vi "Read Marker.vi"(0 "VISA resource name":refnum<visa-resource-name>, 5 "Measurement Type (6: Phase Noise)":u16(ring)=6 items=["AM Noise"=1, "Baseband Noise"=2, "Freq/Power"=3, "Spectrum"=4, "Transient"=5, "Phase Noise"=6, "User"=7], 7 "Select Trace (1: 1)":u16(ring)=1 items=["1"=1, "2"=2, "3"=3, "4"=4, "5"=5, "6"=6, "7"=7, "8"=8], 9 "Select Marker (1: 1)":u16(ring)=1 items=["1"=1, "2"=2, "3"=3, "4"=4, "5"=5, "6"=6, "7"=7, "8"=8, "9"=9, "10"=10], 11 "error in (no error)":errorcluster, 12 "Maximum Time (10000 ms)":u32=10000) -> (4 "VISA resource name out":refnum<visa-resource-name>, 6 "X Position":dbl format="%^#_9g", 10 "Y Position":dbl format="%^#_9g", 15 "error out":errorcluster)   [LabVIEW 2011, in "Agilent E5052X.lvlib"]
doc: "Reads the X and Y positions of the selected marker for the selected trace of the selected measurement. \n\n<b>Note: </b> \n\n\"Configure Marker\" and \"Configure Marker Search\" VIs should be run before calling this VI."
uses:
  Agilent E5052X.lvlib
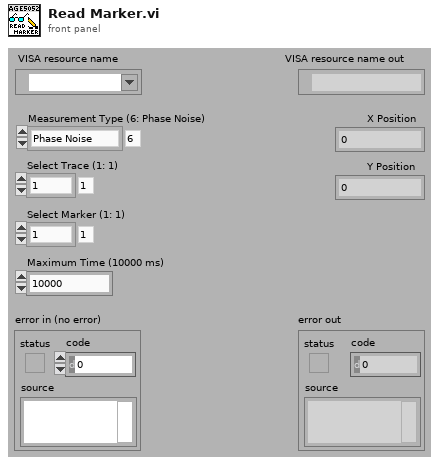
[diagram p1: front panel]
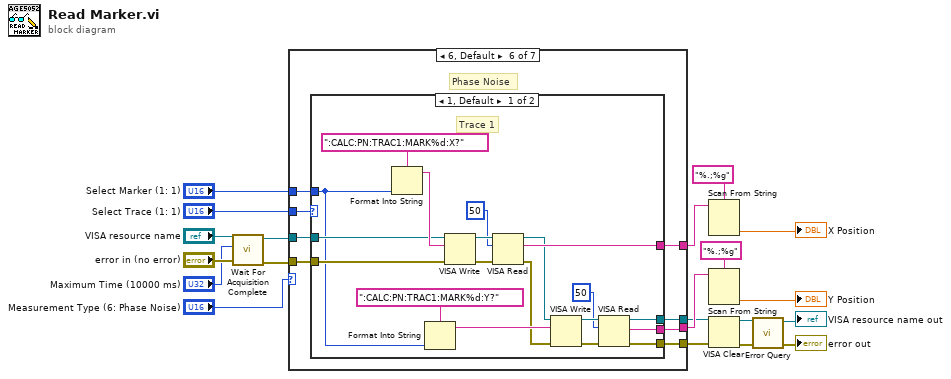
[diagram p0: block diagram]
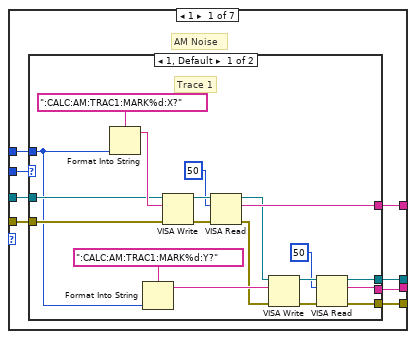
[diagram p2: hidden frame]
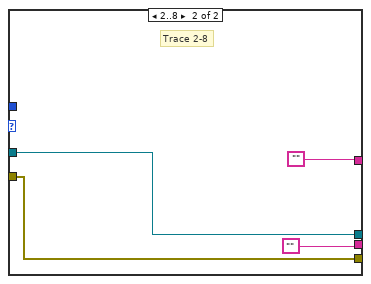
[diagram p3: hidden frame]
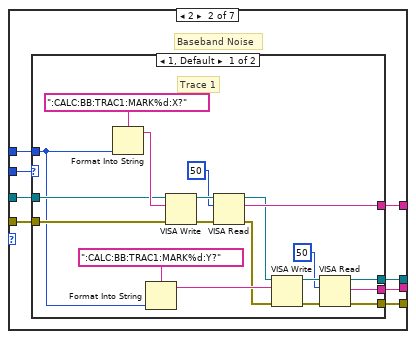
[diagram p4: hidden frame]
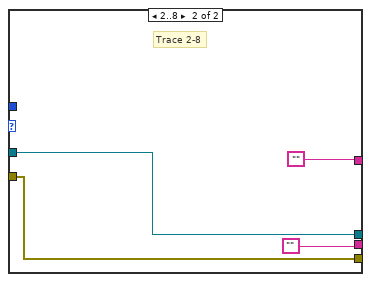
[diagram p5: hidden frame]
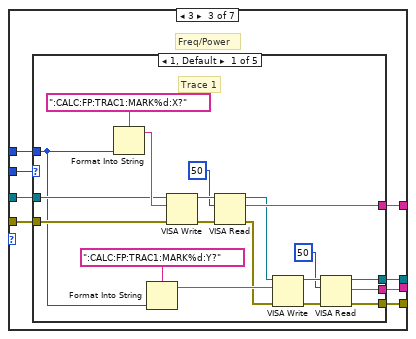
[diagram p6: hidden frame]
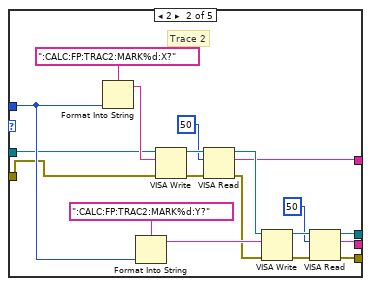
[diagram p7: hidden frame]
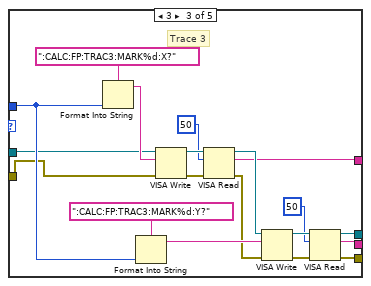
[diagram p8: hidden frame]
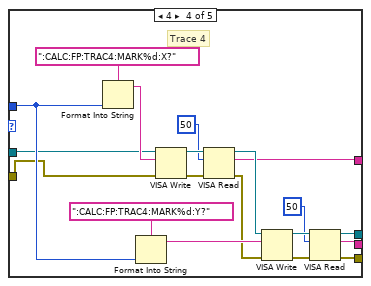
[diagram p9: hidden frame]
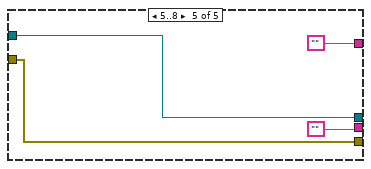
[diagram p10: hidden frame]
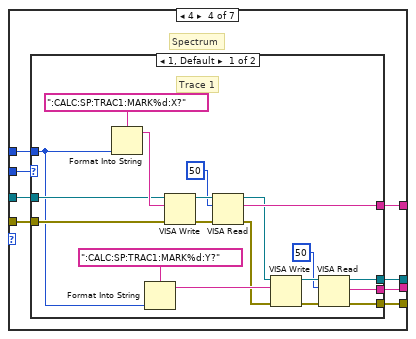
[diagram p11: hidden frame]
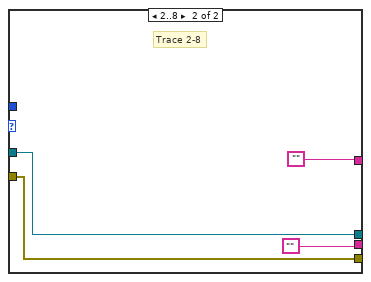
[diagram p12: hidden frame]
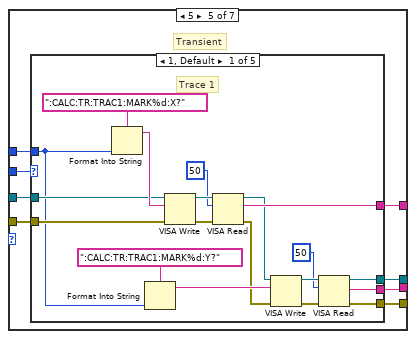
[diagram p13: hidden frame]
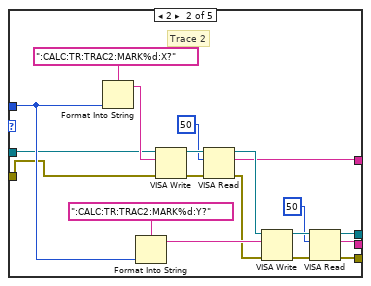
[diagram p14: hidden frame]
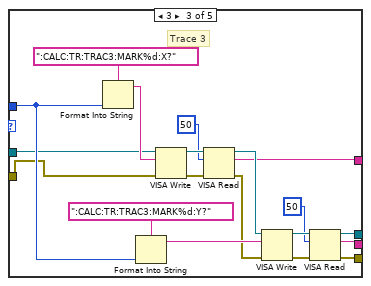
[diagram p15: hidden frame]
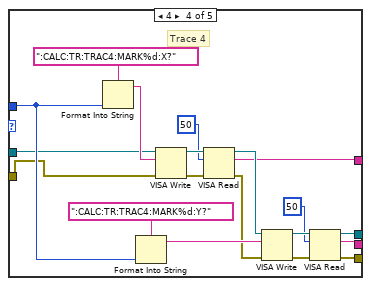
[diagram p16: hidden frame]
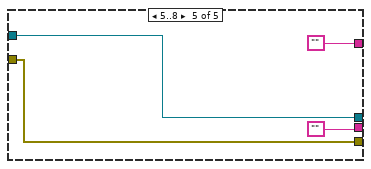
[diagram p17: hidden frame]
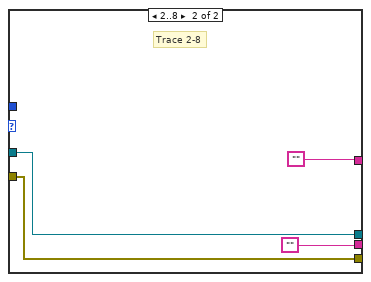
[diagram p18: hidden frame]
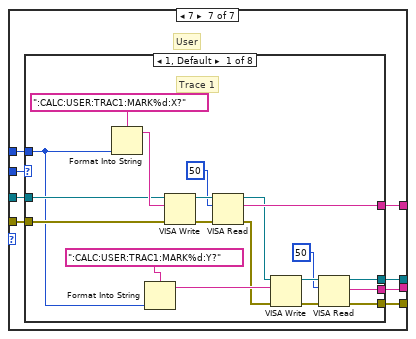
[diagram p19: hidden frame]
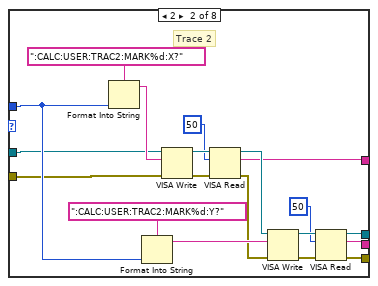
[diagram p20: hidden frame]
diagram:
  n1 = call "Wait For Acquisition Complete.vi"("error in (no error)"="error in (no error)", "Maximum Time (10000)"="Maximum Time (10000 ms)", "VISA resource name"="VISA resource name") -> ("error out"=w7:errorcluster, "VISA resource name out"=w6:refnum<visa-resource-name>)  [unwired: 7 in]
  n2 = case shown="6, Default" "Measurement Type (6: Phase Noise)" {
    tunnel: "Select Trace (1: 1)" -> [w28 w58 w89 w177 w208 w296 w327]
    tunnel: "Select Marker (1: 1)" -> [w27 w59 w90 w178 w209 w297 w328]
    tunnel: w6 -> [w26 w57 w88 w176 w207 w295 w326]
    tunnel: w7 -> [w25 w56 w87 w175 w206 w294 w325]
    tunnel: [w24 w55 w86 w174 w205 w293 w324] -> w18
    tunnel: [w23 w54 w85 w173 w204 w292 w323] -> w11
    tunnel: [w22 w53 w84 w172 w203 w291 w322] -> w15
    tunnel: [w21 w52 w83 w171 w202 w290 w321] -> w10
    frame 1 {
      # "AM Noise"
      n3 = case shown="1, Default" w28 {
        tunnel: w27 -> [w32 _]
        tunnel: w26 -> [w45 w49]
        tunnel: w25 -> [w44 w48]
        tunnel: [w40 ""] -> w24
        tunnel: [w31 w49] -> w23
        tunnel: [w30 ""] -> w22
        tunnel: [w29 w48] -> w21
        frame 1, Default {
          # "Trace 1"
          n4 = Format Into String(format string=":CALC:AM:TRAC1:MARK%d:X?", w32) -> (resulting string=w46:string)  [unwired: 2 in, 1 out]
          n5 = Format Into String(format string=":CALC:AM:TRAC1:MARK%d:Y?", w32) -> (resulting string=w38:string)  [unwired: 2 in, 1 out]
          n6 = VISA Write(VISA resource name=w45, write buffer=w46, error in (no error)=w44) -> (VISA resource name out=w42:refnum<visa-resource-name>, error out=w43:errorcluster)  [unwired: 1 out]
          n7 = VISA Read(VISA resource name=w42, byte count=u32 50, error in (no error)=w43) -> (VISA resource name out=w34:refnum<visa-resource-name>, read buffer=w40:string, error out=w33:errorcluster)  [unwired: 1 out]
          n8 = VISA Write(VISA resource name=w34, write buffer=w38, error in (no error)=w33) -> (VISA resource name out=w36:refnum<visa-resource-name>, error out=w37:errorcluster)  [unwired: 1 out]
          n9 = VISA Read(VISA resource name=w36, byte count=u32 50, error in (no error)=w37) -> (VISA resource name out=w31:refnum<visa-resource-name>, read buffer=w30:string, error out=w29:errorcluster)  [unwired: 1 out]
        }
        frame 2..8 {
          # "Trace 2-8"
        }
      }
    }
    frame 2 {
      # "Baseband Noise"
      n10 = case shown="1, Default" w58 {
        tunnel: w59 -> [w63 _]
        tunnel: w57 -> [w76 w80]
        tunnel: w56 -> [w75 w79]
        tunnel: [w71 ""] -> w55
        tunnel: [w62 w80] -> w54
        tunnel: [w61 ""] -> w53
        tunnel: [w60 w79] -> w52
        frame 1, Default {
          # "Trace 1"
          n11 = Format Into String(format string=":CALC:BB:TRAC1:MARK%d:X?", w63) -> (resulting string=w77:string)  [unwired: 2 in, 1 out]
          n12 = Format Into String(format string=":CALC:BB:TRAC1:MARK%d:Y?", w63) -> (resulting string=w69:string)  [unwired: 2 in, 1 out]
          n13 = VISA Write(VISA resource name=w76, write buffer=w77, error in (no error)=w75) -> (VISA resource name out=w73:refnum<visa-resource-name>, error out=w74:errorcluster)  [unwired: 1 out]
          n14 = VISA Read(VISA resource name=w73, byte count=u32 50, error in (no error)=w74) -> (VISA resource name out=w65:refnum<visa-resource-name>, read buffer=w71:string, error out=w64:errorcluster)  [unwired: 1 out]
          n15 = VISA Write(VISA resource name=w65, write buffer=w69, error in (no error)=w64) -> (VISA resource name out=w67:refnum<visa-resource-name>, error out=w68:errorcluster)  [unwired: 1 out]
          n16 = VISA Read(VISA resource name=w67, byte count=u32 50, error in (no error)=w68) -> (VISA resource name out=w62:refnum<visa-resource-name>, read buffer=w61:string, error out=w60:errorcluster)  [unwired: 1 out]
        }
        frame 2..8 {
          # "Trace 2-8"
        }
      }
    }
    frame 3 {
      # "Freq/Power"
      n17 = case shown="1, Default" w89 {
        tunnel: w90 -> [w94 w116 w135 w154 _]
        tunnel: w88 -> [w107 w115 w134 w153 w168]
        tunnel: w87 -> [w106 w114 w133 w152 w167]
        tunnel: [w102 w113 w132 w151 ""] -> w86
        tunnel: [w93 w112 w131 w150 w168] -> w85
        tunnel: [w92 w111 w130 w149 ""] -> w84
        tunnel: [w91 w110 w129 w148 w167] -> w83
        frame 1, Default {
          # "Trace 1"
          n18 = Format Into String(format string=":CALC:FP:TRAC1:MARK%d:X?", w94) -> (resulting string=w108:string)  [unwired: 2 in, 1 out]
          n19 = Format Into String(format string=":CALC:FP:TRAC1:MARK%d:Y?", w94) -> (resulting string=w100:string)  [unwired: 2 in, 1 out]
          n20 = VISA Write(VISA resource name=w107, write buffer=w108, error in (no error)=w106) -> (VISA resource name out=w104:refnum<visa-resource-name>, error out=w105:errorcluster)  [unwired: 1 out]
          n21 = VISA Read(VISA resource name=w104, byte count=u32 50, error in (no error)=w105) -> (VISA resource name out=w96:refnum<visa-resource-name>, read buffer=w102:string, error out=w95:errorcluster)  [unwired: 1 out]
          n22 = VISA Write(VISA resource name=w96, write buffer=w100, error in (no error)=w95) -> (VISA resource name out=w98:refnum<visa-resource-name>, error out=w99:errorcluster)  [unwired: 1 out]
          n23 = VISA Read(VISA resource name=w98, byte count=u32 50, error in (no error)=w99) -> (VISA resource name out=w93:refnum<visa-resource-name>, read buffer=w92:string, error out=w91:errorcluster)  [unwired: 1 out]
        }
        frame 2 {
          # "Trace 2"
          n24 = Format Into String(format string=":CALC:FP:TRAC2:MARK%d:X?", w116) -> (resulting string=w127:string)  [unwired: 2 in, 1 out]
          n25 = Format Into String(format string=":CALC:FP:TRAC2:MARK%d:Y?", w116) -> (resulting string=w122:string)  [unwired: 2 in, 1 out]
          n26 = VISA Write(VISA resource name=w115, write buffer=w127, error in (no error)=w114) -> (VISA resource name out=w125:refnum<visa-resource-name>, error out=w126:errorcluster)  [unwired: 1 out]
          n27 = VISA Read(VISA resource name=w125, byte count=u32 50, error in (no error)=w126) -> (VISA resource name out=w118:refnum<visa-resource-name>, read buffer=w113:string, error out=w117:errorcluster)  [unwired: 1 out]
          n28 = VISA Write(VISA resource name=w118, write buffer=w122, error in (no error)=w117) -> (VISA resource name out=w120:refnum<visa-resource-name>, error out=w121:errorcluster)  [unwired: 1 out]
          n29 = VISA Read(VISA resource name=w120, byte count=u32 50, error in (no error)=w121) -> (VISA resource name out=w112:refnum<visa-resource-name>, read buffer=w111:string, error out=w110:errorcluster)  [unwired: 1 out]
        }
        frame 3 {
          # "Trace 3"
          n30 = Format Into String(format string=":CALC:FP:TRAC3:MARK%d:X?", w135) -> (resulting string=w146:string)  [unwired: 2 in, 1 out]
          n31 = Format Into String(format string=":CALC:FP:TRAC3:MARK%d:Y?", w135) -> (resulting string=w141:string)  [unwired: 2 in, 1 out]
          n32 = VISA Write(VISA resource name=w134, write buffer=w146, error in (no error)=w133) -> (VISA resource name out=w144:refnum<visa-resource-name>, error out=w145:errorcluster)  [unwired: 1 out]
          n33 = VISA Read(VISA resource name=w144, byte count=u32 50, error in (no error)=w145) -> (VISA resource name out=w137:refnum<visa-resource-name>, read buffer=w132:string, error out=w136:errorcluster)  [unwired: 1 out]
          n34 = VISA Write(VISA resource name=w137, write buffer=w141, error in (no error)=w136) -> (VISA resource name out=w139:refnum<visa-resource-name>, error out=w140:errorcluster)  [unwired: 1 out]
          n35 = VISA Read(VISA resource name=w139, byte count=u32 50, error in (no error)=w140) -> (VISA resource name out=w131:refnum<visa-resource-name>, read buffer=w130:string, error out=w129:errorcluster)  [unwired: 1 out]
        }
        frame 4 {
          # "Trace 4"
          n36 = Format Into String(format string=":CALC:FP:TRAC4:MARK%d:X?", w154) -> (resulting string=w165:string)  [unwired: 2 in, 1 out]
          n37 = Format Into String(format string=":CALC:FP:TRAC4:MARK%d:Y?", w154) -> (resulting string=w160:string)  [unwired: 2 in, 1 out]
          n38 = VISA Write(VISA resource name=w153, write buffer=w165, error in (no error)=w152) -> (VISA resource name out=w163:refnum<visa-resource-name>, error out=w164:errorcluster)  [unwired: 1 out]
          n39 = VISA Read(VISA resource name=w163, byte count=u32 50, error in (no error)=w164) -> (VISA resource name out=w156:refnum<visa-resource-name>, read buffer=w151:string, error out=w155:errorcluster)  [unwired: 1 out]
          n40 = VISA Write(VISA resource name=w156, write buffer=w160, error in (no error)=w155) -> (VISA resource name out=w158:refnum<visa-resource-name>, error out=w159:errorcluster)  [unwired: 1 out]
          n41 = VISA Read(VISA resource name=w158, byte count=u32 50, error in (no error)=w159) -> (VISA resource name out=w150:refnum<visa-resource-name>, read buffer=w149:string, error out=w148:errorcluster)  [unwired: 1 out]
        }
        frame 5..8 {
        }
      }
    }
    frame 4 {
      # "Spectrum"
      n42 = case shown="1, Default" w177 {
        tunnel: w178 -> [w182 _]
        tunnel: w176 -> [w195 w199]
        tunnel: w175 -> [w194 w198]
        tunnel: [w190 ""] -> w174
        tunnel: [w181 w199] -> w173
        tunnel: [w180 ""] -> w172
        tunnel: [w179 w198] -> w171
        frame 1, Default {
          # "Trace 1"
          n43 = Format Into String(format string=":CALC:SP:TRAC1:MARK%d:X?", w182) -> (resulting string=w196:string)  [unwired: 2 in, 1 out]
          n44 = Format Into String(format string=":CALC:SP:TRAC1:MARK%d:Y?", w182) -> (resulting string=w188:string)  [unwired: 2 in, 1 out]
          n45 = VISA Write(VISA resource name=w195, write buffer=w196, error in (no error)=w194) -> (VISA resource name out=w192:refnum<visa-resource-name>, error out=w193:errorcluster)  [unwired: 1 out]
          n46 = VISA Read(VISA resource name=w192, byte count=u32 50, error in (no error)=w193) -> (VISA resource name out=w184:refnum<visa-resource-name>, read buffer=w190:string, error out=w183:errorcluster)  [unwired: 1 out]
          n47 = VISA Write(VISA resource name=w184, write buffer=w188, error in (no error)=w183) -> (VISA resource name out=w186:refnum<visa-resource-name>, error out=w187:errorcluster)  [unwired: 1 out]
          n48 = VISA Read(VISA resource name=w186, byte count=u32 50, error in (no error)=w187) -> (VISA resource name out=w181:refnum<visa-resource-name>, read buffer=w180:string, error out=w179:errorcluster)  [unwired: 1 out]
        }
        frame 2..8 {
          # "Trace 2-8"
        }
      }
    }
    frame 5 {
      # "Transient"
      n49 = case shown="1, Default" w208 {
        tunnel: w209 -> [w213 w235 w254 w273 _]
        tunnel: w207 -> [w226 w234 w253 w272 w287]
        tunnel: w206 -> [w225 w233 w252 w271 w286]
        tunnel: [w221 w232 w251 w270 ""] -> w205
        tunnel: [w212 w231 w250 w269 w287] -> w204
        tunnel: [w211 w230 w249 w268 ""] -> w203
        tunnel: [w210 w229 w248 w267 w286] -> w202
        frame 1, Default {
          # "Trace 1"
          n50 = Format Into String(format string=":CALC:TR:TRAC1:MARK%d:X?", w213) -> (resulting string=w227:string)  [unwired: 2 in, 1 out]
          n51 = Format Into String(format string=":CALC:TR:TRAC1:MARK%d:Y?", w213) -> (resulting string=w219:string)  [unwired: 2 in, 1 out]
          n52 = VISA Write(VISA resource name=w226, write buffer=w227, error in (no error)=w225) -> (VISA resource name out=w223:refnum<visa-resource-name>, error out=w224:errorcluster)  [unwired: 1 out]
          n53 = VISA Read(VISA resource name=w223, byte count=u32 50, error in (no error)=w224) -> (VISA resource name out=w215:refnum<visa-resource-name>, read buffer=w221:string, error out=w214:errorcluster)  [unwired: 1 out]
          n54 = VISA Write(VISA resource name=w215, write buffer=w219, error in (no error)=w214) -> (VISA resource name out=w217:refnum<visa-resource-name>, error out=w218:errorcluster)  [unwired: 1 out]
          n55 = VISA Read(VISA resource name=w217, byte count=u32 50, error in (no error)=w218) -> (VISA resource name out=w212:refnum<visa-resource-name>, read buffer=w211:string, error out=w210:errorcluster)  [unwired: 1 out]
        }
        frame 2 {
          # "Trace 2"
          n56 = Format Into String(format string=":CALC:TR:TRAC2:MARK%d:X?", w235) -> (resulting string=w246:string)  [unwired: 2 in, 1 out]
          n57 = Format Into String(format string=":CALC:TR:TRAC2:MARK%d:Y?", w235) -> (resulting string=w241:string)  [unwired: 2 in, 1 out]
          n58 = VISA Write(VISA resource name=w234, write buffer=w246, error in (no error)=w233) -> (VISA resource name out=w244:refnum<visa-resource-name>, error out=w245:errorcluster)  [unwired: 1 out]
          n59 = VISA Read(VISA resource name=w244, byte count=u32 50, error in (no error)=w245) -> (VISA resource name out=w237:refnum<visa-resource-name>, read buffer=w232:string, error out=w236:errorcluster)  [unwired: 1 out]
          n60 = VISA Write(VISA resource name=w237, write buffer=w241, error in (no error)=w236) -> (VISA resource name out=w239:refnum<visa-resource-name>, error out=w240:errorcluster)  [unwired: 1 out]
          n61 = VISA Read(VISA resource name=w239, byte count=u32 50, error in (no error)=w240) -> (VISA resource name out=w231:refnum<visa-resource-name>, read buffer=w230:string, error out=w229:errorcluster)  [unwired: 1 out]
        }
        frame 3 {
          # "Trace 3"
          n62 = Format Into String(format string=":CALC:TR:TRAC3:MARK%d:X?", w254) -> (resulting string=w265:string)  [unwired: 2 in, 1 out]
          n63 = Format Into String(format string=":CALC:TR:TRAC3:MARK%d:Y?", w254) -> (resulting string=w260:string)  [unwired: 2 in, 1 out]
          n64 = VISA Write(VISA resource name=w253, write buffer=w265, error in (no error)=w252) -> (VISA resource name out=w263:refnum<visa-resource-name>, error out=w264:errorcluster)  [unwired: 1 out]
          n65 = VISA Read(VISA resource name=w263, byte count=u32 50, error in (no error)=w264) -> (VISA resource name out=w256:refnum<visa-resource-name>, read buffer=w251:string, error out=w255:errorcluster)  [unwired: 1 out]
          n66 = VISA Write(VISA resource name=w256, write buffer=w260, error in (no error)=w255) -> (VISA resource name out=w258:refnum<visa-resource-name>, error out=w259:errorcluster)  [unwired: 1 out]
          n67 = VISA Read(VISA resource name=w258, byte count=u32 50, error in (no error)=w259) -> (VISA resource name out=w250:refnum<visa-resource-name>, read buffer=w249:string, error out=w248:errorcluster)  [unwired: 1 out]
        }
        frame 4 {
          # "Trace 4"
          n68 = Format Into String(format string=":CALC:TR:TRAC4:MARK%d:X?", w273) -> (resulting string=w284:string)  [unwired: 2 in, 1 out]
          n69 = Format Into String(format string=":CALC:TR:TRAC4:MARK%d:Y?", w273) -> (resulting string=w279:string)  [unwired: 2 in, 1 out]
          n70 = VISA Write(VISA resource name=w272, write buffer=w284, error in (no error)=w271) -> (VISA resource name out=w282:refnum<visa-resource-name>, error out=w283:errorcluster)  [unwired: 1 out]
          n71 = VISA Read(VISA resource name=w282, byte count=u32 50, error in (no error)=w283) -> (VISA resource name out=w275:refnum<visa-resource-name>, read buffer=w270:string, error out=w274:errorcluster)  [unwired: 1 out]
          n72 = VISA Write(VISA resource name=w275, write buffer=w279, error in (no error)=w274) -> (VISA resource name out=w277:refnum<visa-resource-name>, error out=w278:errorcluster)  [unwired: 1 out]
          n73 = VISA Read(VISA resource name=w277, byte count=u32 50, error in (no error)=w278) -> (VISA resource name out=w269:refnum<visa-resource-name>, read buffer=w268:string, error out=w267:errorcluster)  [unwired: 1 out]
        }
        frame 5..8 {
        }
      }
    }
    frame 6, Default {
      # "Phase Noise"
      n74 = case shown="1, Default" w296 {
        tunnel: w297 -> [w301 _]
        tunnel: w295 -> [w314 w318]
        tunnel: w294 -> [w313 w317]
        tunnel: [w309 ""] -> w293
        tunnel: [w300 w318] -> w292
        tunnel: [w299 ""] -> w291
        tunnel: [w298 w317] -> w290
        frame 1, Default {
          # "Trace 1"
          n75 = Format Into String(format string=":CALC:PN:TRAC1:MARK%d:X?", w301) -> (resulting string=w315:string)  [unwired: 2 in, 1 out]
          n76 = Format Into String(format string=":CALC:PN:TRAC1:MARK%d:Y?", w301) -> (resulting string=w307:string)  [unwired: 2 in, 1 out]
          n77 = VISA Write(VISA resource name=w314, write buffer=w315, error in (no error)=w313) -> (VISA resource name out=w311:refnum<visa-resource-name>, error out=w312:errorcluster)  [unwired: 1 out]
          n78 = VISA Read(VISA resource name=w311, byte count=u32 50, error in (no error)=w312) -> (VISA resource name out=w303:refnum<visa-resource-name>, read buffer=w309:string, error out=w302:errorcluster)  [unwired: 1 out]
          n79 = VISA Write(VISA resource name=w303, write buffer=w307, error in (no error)=w302) -> (VISA resource name out=w305:refnum<visa-resource-name>, error out=w306:errorcluster)  [unwired: 1 out]
          n80 = VISA Read(VISA resource name=w305, byte count=u32 50, error in (no error)=w306) -> (VISA resource name out=w300:refnum<visa-resource-name>, read buffer=w299:string, error out=w298:errorcluster)  [unwired: 1 out]
        }
        frame 2..8 {
          # "Trace 2-8"
        }
      }
    }
    frame 7 {
      # "User"
      n81 = case shown="1, Default" w327 {
        tunnel: w328 -> [w332 w354 w373 w392 w411 w430 w449 w468]
        tunnel: w326 -> [w345 w353 w372 w391 w410 w429 w448 w467]
        tunnel: w325 -> [w344 w352 w371 w390 w409 w428 w447 w466]
        tunnel: [w340 w351 w370 w389 w408 w427 w446 w465] -> w324
        tunnel: [w331 w350 w369 w388 w407 w426 w445 w464] -> w323
        tunnel: [w330 w349 w368 w387 w406 w424 w443 w463] -> w322
        tunnel: [w329 w348 w367 w386 w405 w425 w444 w462] -> w321
        frame 1, Default {
          # "Trace 1"
          n82 = Format Into String(format string=":CALC:USER:TRAC1:MARK%d:X?", w332) -> (resulting string=w346:string)  [unwired: 2 in, 1 out]
          n83 = Format Into String(format string=":CALC:USER:TRAC1:MARK%d:Y?", w332) -> (resulting string=w338:string)  [unwired: 2 in, 1 out]
          n84 = VISA Write(VISA resource name=w345, write buffer=w346, error in (no error)=w344) -> (VISA resource name out=w342:refnum<visa-resource-name>, error out=w343:errorcluster)  [unwired: 1 out]
          n85 = VISA Read(VISA resource name=w342, byte count=u32 50, error in (no error)=w343) -> (VISA resource name out=w334:refnum<visa-resource-name>, read buffer=w340:string, error out=w333:errorcluster)  [unwired: 1 out]
          n86 = VISA Write(VISA resource name=w334, write buffer=w338, error in (no error)=w333) -> (VISA resource name out=w336:refnum<visa-resource-name>, error out=w337:errorcluster)  [unwired: 1 out]
          n87 = VISA Read(VISA resource name=w336, byte count=u32 50, error in (no error)=w337) -> (VISA resource name out=w331:refnum<visa-resource-name>, read buffer=w330:string, error out=w329:errorcluster)  [unwired: 1 out]
        }
        frame 2 {
          # "Trace 2"
          n88 = Format Into String(format string=":CALC:USER:TRAC2:MARK%d:X?", w354) -> (resulting string=w365:string)  [unwired: 2 in, 1 out]
          n89 = Format Into String(format string=":CALC:USER:TRAC2:MARK%d:Y?", w354) -> (resulting string=w360:string)  [unwired: 2 in, 1 out]
          n90 = VISA Write(VISA resource name=w353, write buffer=w365, error in (no error)=w352) -> (VISA resource name out=w363:refnum<visa-resource-name>, error out=w364:errorcluster)  [unwired: 1 out]
          n91 = VISA Read(VISA resource name=w363, byte count=u32 50, error in (no error)=w364) -> (VISA resource name out=w356:refnum<visa-resource-name>, read buffer=w351:string, error out=w355:errorcluster)  [unwired: 1 out]
          n92 = VISA Write(VISA resource name=w356, write buffer=w360, error in (no error)=w355) -> (VISA resource name out=w358:refnum<visa-resource-name>, error out=w359:errorcluster)  [unwired: 1 out]
          n93 = VISA Read(VISA resource name=w358, byte count=u32 50, error in (no error)=w359) -> (VISA resource name out=w350:refnum<visa-resource-name>, read buffer=w349:string, error out=w348:errorcluster)  [unwired: 1 out]
        }
        frame 3 {
          # "Trace 3"
          n94 = Format Into String(format string=":CALC:USER:TRAC3:MARK%d:X?", w373) -> (resulting string=w384:string)  [unwired: 2 in, 1 out]
          n95 = Format Into String(format string=":CALC:USER:TRAC3:MARK%d:Y?", w373) -> (resulting string=w379:string)  [unwired: 2 in, 1 out]
          n96 = VISA Write(VISA resource name=w372, write buffer=w384, error in (no error)=w371) -> (VISA resource name out=w382:refnum<visa-resource-name>, error out=w383:errorcluster)  [unwired: 1 out]
          n97 = VISA Read(VISA resource name=w382, byte count=u32 50, error in (no error)=w383) -> (VISA resource name out=w375:refnum<visa-resource-name>, read buffer=w370:string, error out=w374:errorcluster)  [unwired: 1 out]
          n98 = VISA Write(VISA resource name=w375, write buffer=w379, error in (no error)=w374) -> (VISA resource name out=w377:refnum<visa-resource-name>, error out=w378:errorcluster)  [unwired: 1 out]
          n99 = VISA Read(VISA resource name=w377, byte count=u32 50, error in (no error)=w378) -> (VISA resource name out=w369:refnum<visa-resource-name>, read buffer=w368:string, error out=w367:errorcluster)  [unwired: 1 out]
        }
        frame 4 {
          # "Trace 4"
          n100 = Format Into String(format string=":CALC:USER:TRAC4:MARK%d:X?", w392) -> (resulting string=w403:string)  [unwired: 2 in, 1 out]
          n101 = Format Into String(format string=":CALC:USER:TRAC4:MARK%d:Y?", w392) -> (resulting string=w398:string)  [unwired: 2 in, 1 out]
          n102 = VISA Write(VISA resource name=w391, write buffer=w403, error in (no error)=w390) -> (VISA resource name out=w401:refnum<visa-resource-name>, error out=w402:errorcluster)  [unwired: 1 out]
          n103 = VISA Read(VISA resource name=w401, byte count=u32 50, error in (no error)=w402) -> (VISA resource name out=w394:refnum<visa-resource-name>, read buffer=w389:string, error out=w393:errorcluster)  [unwired: 1 out]
          n104 = VISA Write(VISA resource name=w394, write buffer=w398, error in (no error)=w393) -> (VISA resource name out=w396:refnum<visa-resource-name>, error out=w397:errorcluster)  [unwired: 1 out]
          n105 = VISA Read(VISA resource name=w396, byte count=u32 50, error in (no error)=w397) -> (VISA resource name out=w388:refnum<visa-resource-name>, read buffer=w387:string, error out=w386:errorcluster)  [unwired: 1 out]
        }
        frame 5 {
          # "Trace 5"
          n106 = Format Into String(format string=":CALC:USER:TRAC5:MARK%d:X?", w411) -> (resulting string=w422:string)  [unwired: 2 in, 1 out]
          n107 = Format Into String(format string=":CALC:USER:TRAC5:MARK%d:Y?", w411) -> (resulting string=w417:string)  [unwired: 2 in, 1 out]
          n108 = VISA Write(VISA resource name=w410, write buffer=w422, error in (no error)=w409) -> (VISA resource name out=w420:refnum<visa-resource-name>, error out=w421:errorcluster)  [unwired: 1 out]
          n109 = VISA Read(VISA resource name=w420, byte count=u32 50, error in (no error)=w421) -> (VISA resource name out=w413:refnum<visa-resource-name>, read buffer=w408:string, error out=w412:errorcluster)  [unwired: 1 out]
          n110 = VISA Write(VISA resource name=w413, write buffer=w417, error in (no error)=w412) -> (VISA resource name out=w415:refnum<visa-resource-name>, error out=w416:errorcluster)  [unwired: 1 out]
          n111 = VISA Read(VISA resource name=w415, byte count=u32 50, error in (no error)=w416) -> (VISA resource name out=w407:refnum<visa-resource-name>, read buffer=w406:string, error out=w405:errorcluster)  [unwired: 1 out]
        }
        frame 6 {
          # "Trace 6"
          n112 = Format Into String(format string=":CALC:USER:TRAC6:MARK%d:X?", w430) -> (resulting string=w441:string)  [unwired: 2 in, 1 out]
          n113 = Format Into String(format string=":CALC:USER:TRAC6:MARK%d:Y?", w430) -> (resulting string=w436:string)  [unwired: 2 in, 1 out]
          n114 = VISA Write(VISA resource name=w429, write buffer=w441, error in (no error)=w428) -> (VISA resource name out=w439:refnum<visa-resource-name>, error out=w440:errorcluster)  [unwired: 1 out]
          n115 = VISA Read(VISA resource name=w439, byte count=u32 50, error in (no error)=w440) -> (VISA resource name out=w432:refnum<visa-resource-name>, read buffer=w427:string, error out=w431:errorcluster)  [unwired: 1 out]
          n116 = VISA Write(VISA resource name=w432, write buffer=w436, error in (no error)=w431) -> (VISA resource name out=w434:refnum<visa-resource-name>, error out=w435:errorcluster)  [unwired: 1 out]
          n117 = VISA Read(VISA resource name=w434, byte count=u32 50, error in (no error)=w435) -> (VISA resource name out=w426:refnum<visa-resource-name>, read buffer=w424:string, error out=w425:errorcluster)  [unwired: 1 out]
        }
        frame 7 {
          # "Trace 7"
          n118 = Format Into String(format string=":CALC:USER:TRAC7:MARK%d:X?", w449) -> (resulting string=w460:string)  [unwired: 2 in, 1 out]
          n119 = Format Into String(format string=":CALC:USER:TRAC7:MARK%d:Y?", w449) -> (resulting string=w455:string)  [unwired: 2 in, 1 out]
          n120 = VISA Write(VISA resource name=w448, write buffer=w460, error in (no error)=w447) -> (VISA resource name out=w458:refnum<visa-resource-name>, error out=w459:errorcluster)  [unwired: 1 out]
          n121 = VISA Read(VISA resource name=w458, byte count=u32 50, error in (no error)=w459) -> (VISA resource name out=w451:refnum<visa-resource-name>, read buffer=w446:string, error out=w450:errorcluster)  [unwired: 1 out]
          n122 = VISA Write(VISA resource name=w451, write buffer=w455, error in (no error)=w450) -> (VISA resource name out=w453:refnum<visa-resource-name>, error out=w454:errorcluster)  [unwired: 1 out]
          n123 = VISA Read(VISA resource name=w453, byte count=u32 50, error in (no error)=w454) -> (VISA resource name out=w445:refnum<visa-resource-name>, read buffer=w443:string, error out=w444:errorcluster)  [unwired: 1 out]
        }
        frame 8 {
          # "Trace 8"
          n124 = Format Into String(format string=":CALC:USER:TRAC8:MARK%d:X?", w468) -> (resulting string=w479:string)  [unwired: 2 in, 1 out]
          n125 = Format Into String(format string=":CALC:USER:TRAC8:MARK%d:Y?", w468) -> (resulting string=w474:string)  [unwired: 2 in, 1 out]
          n126 = VISA Write(VISA resource name=w467, write buffer=w479, error in (no error)=w466) -> (VISA resource name out=w477:refnum<visa-resource-name>, error out=w478:errorcluster)  [unwired: 1 out]
          n127 = VISA Read(VISA resource name=w477, byte count=u32 50, error in (no error)=w478) -> (VISA resource name out=w470:refnum<visa-resource-name>, read buffer=w465:string, error out=w469:errorcluster)  [unwired: 1 out]
          n128 = VISA Write(VISA resource name=w470, write buffer=w474, error in (no error)=w469) -> (VISA resource name out=w472:refnum<visa-resource-name>, error out=w473:errorcluster)  [unwired: 1 out]
          n129 = VISA Read(VISA resource name=w472, byte count=u32 50, error in (no error)=w473) -> (VISA resource name out=w464:refnum<visa-resource-name>, read buffer=w463:string, error out=w462:errorcluster)  [unwired: 1 out]
        }
      }
    }
  }
  n130 = Scan From String(format string="%.;%g", input string=w18) -> (output 1=→"X Position":dbl)  [unwired: 3 in, 3 out]
  n131 = Scan From String(format string="%.;%g", input string=w15) -> (output 1=→"Y Position":dbl)  [unwired: 3 in, 3 out]
  n132 = VISA Clear(VISA resource name=w11, error in (no error)=w10) -> (VISA resource name out=w2:refnum<visa-resource-name>, error out=w1:errorcluster)
  n133 = call "Error Query.vi"("error in (no error)"=w1, "VISA resource name"=w2) -> ("error out"=→"error out":errorcluster, "VISA resource name out"=→"VISA resource name out":refnum<visa-resource-name>)  [unwired: 6 in, 2 out]
